vi "Get_Sweep_Mode.vi"(8 "error in (no error)":errorcluster, 11 ".NET Reference in":refnum<k24>) -> (0 "error out":errorcluster, 2 "smod":T1(ring), 3 ".NET Reference out":refnum<k24>)   [LabVIEW 2017]
uses:
  LV_IL_Sample/DLL/InstrumentDLL.dll
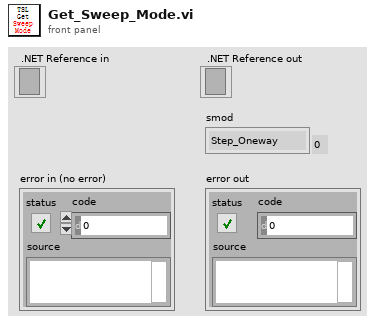
[diagram p1: front panel]
types:
  T1 = enum16{"Step_Oneway", "Continuous_Oneway", "Step_Twoway", "Continuous_Twoway", ""}
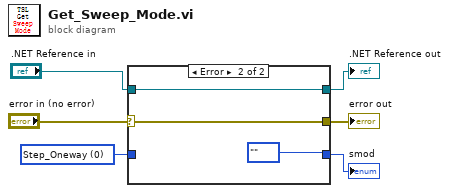
[diagram p0: block diagram]
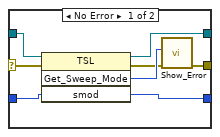
[diagram p2: hidden frame]
diagram:
  w2 = 0 items=["Step_Oneway", "Continuous_Oneway", "Step_Twoway", "Continuous_Twoway"] ("smod")
  n1 = case shown="Error" "error in (no error)" {
    selector: "error in (no error)" -> [w7 w17]
    tunnel: [w8 w17] -> w6
    tunnel: [w14 w16] -> w5
    tunnel: [w13 T1."" ("smod")] -> w4
    tunnel: ".NET Reference in" -> [w12 w16]
    tunnel: w2 -> [w11 _]
    frame No Error {
      n2 = invoke on="调用节点" class="TSL" method="Get_Sweep_Mode"(reference=w12, error in=w7, "smod"=w11) -> (reference out=w14:refnum<k24>, error out=w9:errorcluster, "Get_Sweep_Mode"=w10:i32, "smod"=w13:i32)  [unwired: 1 in]
      n3 = call "Show_Error.vi"("error in (no error)"=w9, "Error"=w10) -> ("error out"=w8:errorcluster)  [unwired: 9 in]
    }
    frame Error {
    }
  }
  "error out" <- w6
  ".NET Reference out" <- w5
  "smod" <- w4
